vi "ClientSDO_Init.vi"(8 "error in (no error)":errorcluster) -> (0 "error out":errorcluster, 3 "ClientSDO Ref out":refnum<k24>)   [LabVIEW 2015, in "CANOpen.lvlib"]
doc: "initialize library for CANOpen ClientSDO"
uses:
  CANOpen.lvlib
  \\Mac\Home/Desktop/imt_test_app 28-06-2012/canopenlib_cli.dll
  canopenlib_cli.dll
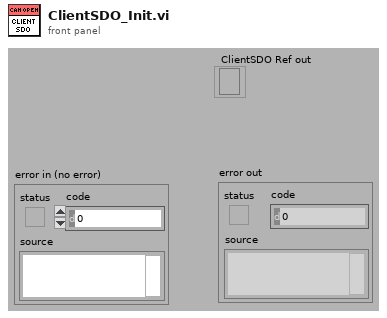
[diagram p1: front panel]
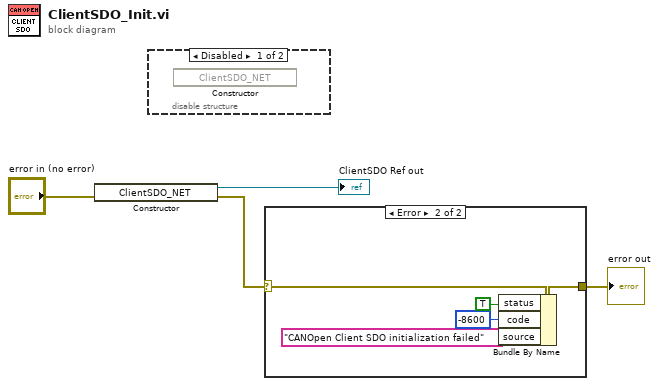
[diagram p0: block diagram]
diagram:
  n1 = constructor class="ClientSDO_NET"(error in="error in (no error)") -> (reference out=→"ClientSDO Ref out":refnum<k24>, error out=w2:errorcluster)  [unwired: 2 in, 1 out]
  n2 = disable-structure shown="Disabled" {
    frame Disabled {
      n3 = constructor class="ClientSDO_NET"() -> ()  [unwired: 3 in, 3 out]
    }
    frame Enabled {
    }
  }
  n4 = case shown="Error" w2 {
    selector: w2 -> [w5 w10]
    tunnel: [w5 w9] -> w4
    frame No Error {
    }
    frame Error {
      n5 = Bundle By Name(cluster=w10, "status"=TRUE, "code"=-8600, "source"="CANOpen Client SDO initialization failed") -> (w9:errorcluster)
    }
  }
  "error out" <- w4
